vi "Turn Left.vi"   [LabVIEW 2011]
uses:
  _GlobalVariables&Libraries/ATV Program Global Variables.vi
types:
  T1 = cluster{"Navigation Coordinates":cluster{"Latitude":dbl, "Longitude":dbl}[], "Coordinate Count":u32, "Drive Speed":string, "Steer Angle":dbl, "Steering":dbl, "Direction to next Coordinate":dbl, "Drive":dbl, "Navigation Path":string}
  T2 = cluster{"Drive Value Output String":string, "Steer Value Output String":string, "Error Out":errorcluster, "Initial Encoder Counts":string, "Disable Galil Terminal":bool, "Command Input":string}
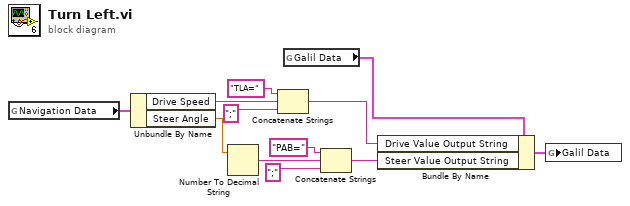
[diagram p0: block diagram]
diagram:
  n1 = global read "ATV Program Global Variables.vi" "Navigation Data"() -> (w4:T1)
  n2 = Unbundle By Name(w4) -> ("Drive Speed"=w3:string, "Steer Angle"=w2:dbl)
  n3 = Number To Decimal String(number=w2) -> (decimal integer string=w1:string)  [unwired: 1 in]
  n4 = Concatenate Strings("TLA=" ("Drive Value Output String"), w3, ";" ("string")) -> (w6:string)
  n5 = global read "ATV Program Global Variables.vi" "Galil Data"() -> (w11:T2)
  n6 = Concatenate Strings("PAB=" ("Drive Value Output String"), w1, ";" ("string")) -> (w5:string)
  n7 = Bundle By Name(cluster=w11, "Drive Value Output String"=w6, "Steer Value Output String"=w5) -> (w12:T2)
  n8 = global write "ATV Program Global Variables.vi" "Galil Data"(w12) -> ()
